vi "Unflatten.vi"(0 "Executioner in":refnum<class "Executioner.lvclass">, 1 "Linked List Ref":refnum<data-value>, 5 "Flattened Test Executive":string, 9 "Linked List ID":string, 11 "error in (no error)":errorcluster, 12 "Persistence in":refnum<class "IPersist.lvclass">, 13 "Compatibility Helper":refnum<class "ICompatibility Helper.lvclass">, 14 "Path Builder":refnum<class "IPath Builder.lvclass">) -> (3 "Linked List Ref out":refnum<data-value>, 6 "Flattened Test Executive out":string, 15 "error out":errorcluster)   [LabVIEW 2020, in "Test Executive.lvlib" / "Executioner.lvclass"]
uses:
  <vilib>/gpm_packages/@cs/test-executive/Source/Test Executive/Executioner/Executioner.lvclass
  <vilib>/gpm_packages/@cs/persistence/source/IPersist/IPersist.lvclass
  <vilib>/gpm_packages/@cs/linked-list/Source/Linked List/ILinkedList/ILinked List.lvclass
  <vilib>/gpm_packages/@cs/test-executive/Source/Path Builder/IPath Builder/IPath Builder.lvclass
  <vilib>/gpm_packages/@cs/test-executive/Source/Compatibility Helper/ICompatibility Helper.lvclass
  7496b3ab-09a6-44dc-ae9e-1065b628b99e.vi
  <vilib>/Utility/error.llb/Error Cluster From Error Code.vi
  <vilib>/ErrorRing/Error Ring.xnode
  <vilib>/gpm_packages/@cs/linked-list/Source/Linked List/Linked List Ref/Linked List Ref.lvclass
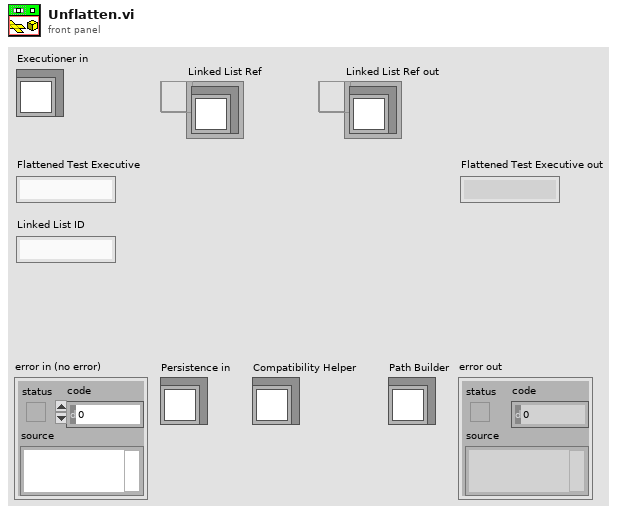
[diagram p1: front panel]
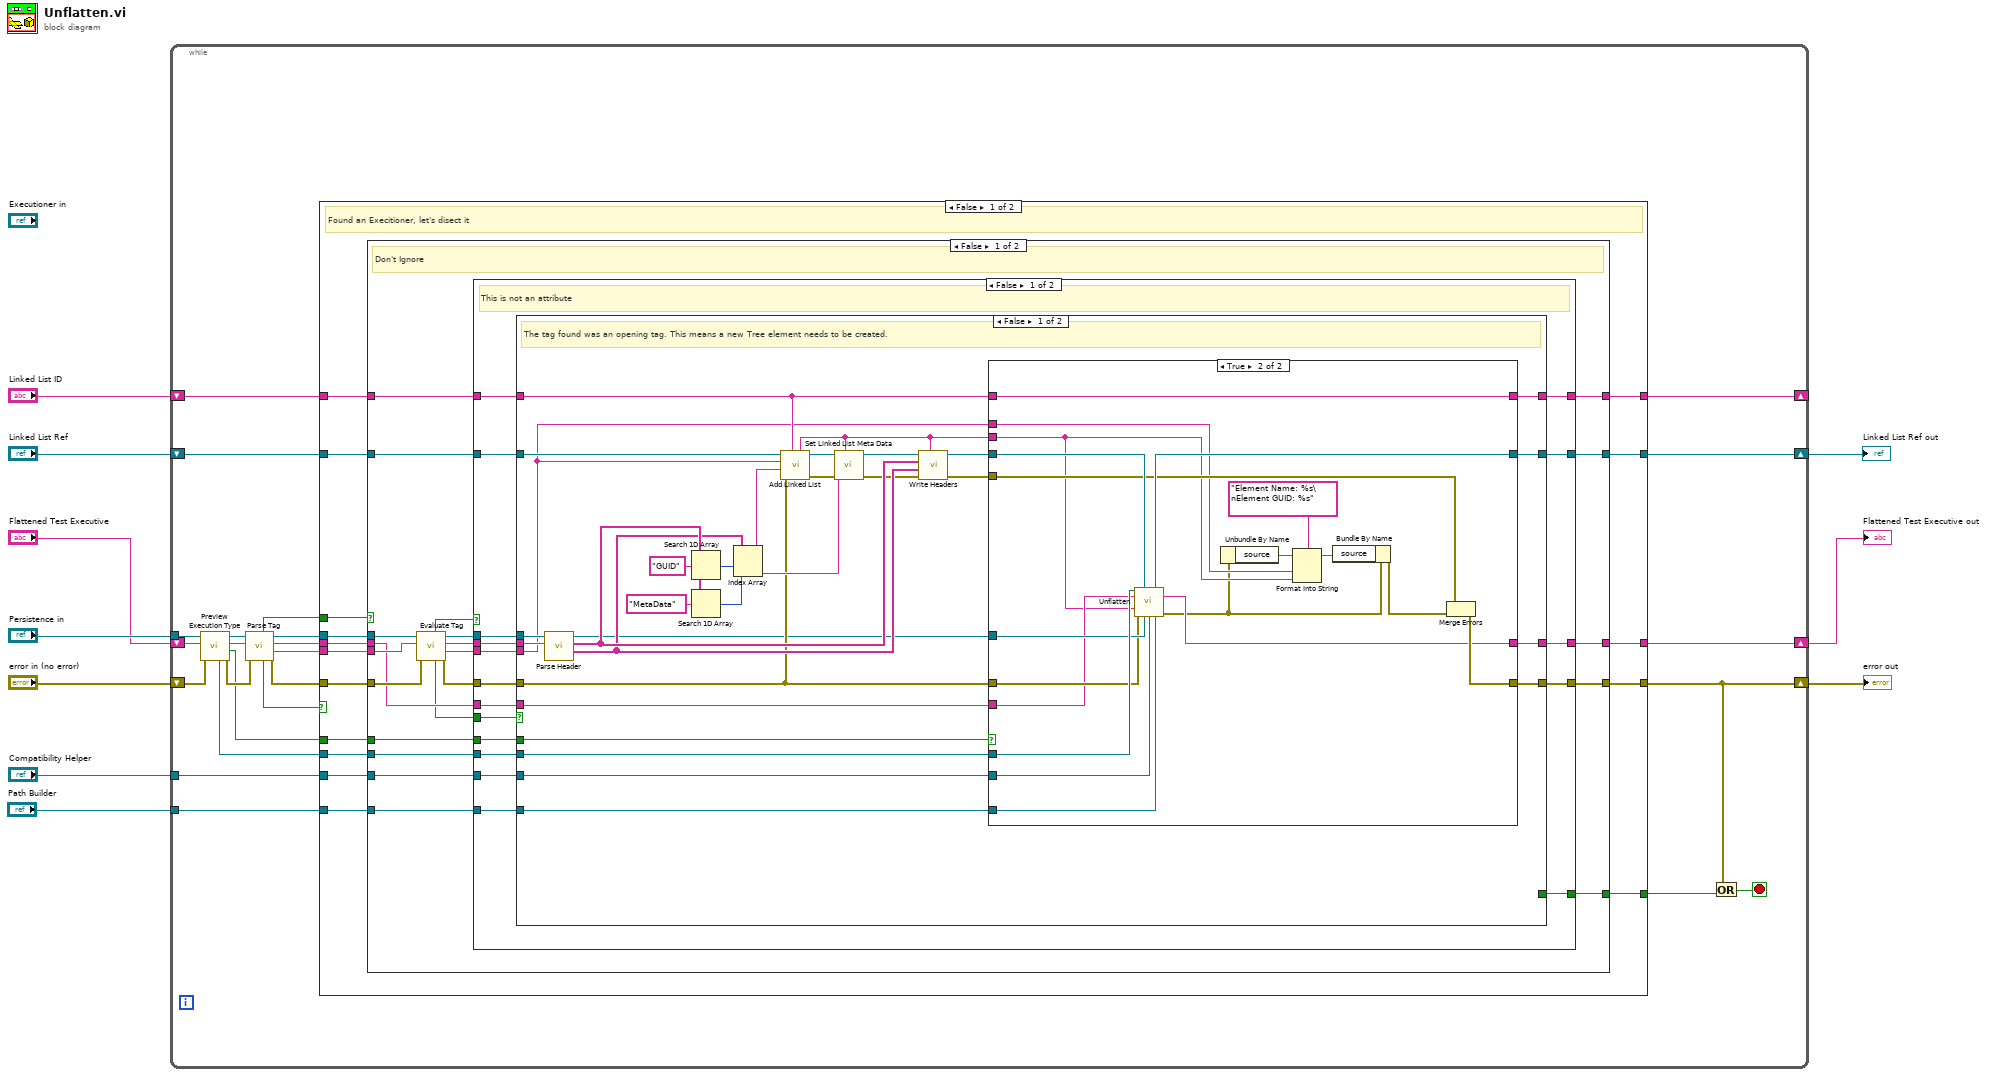
[diagram p0: block diagram]
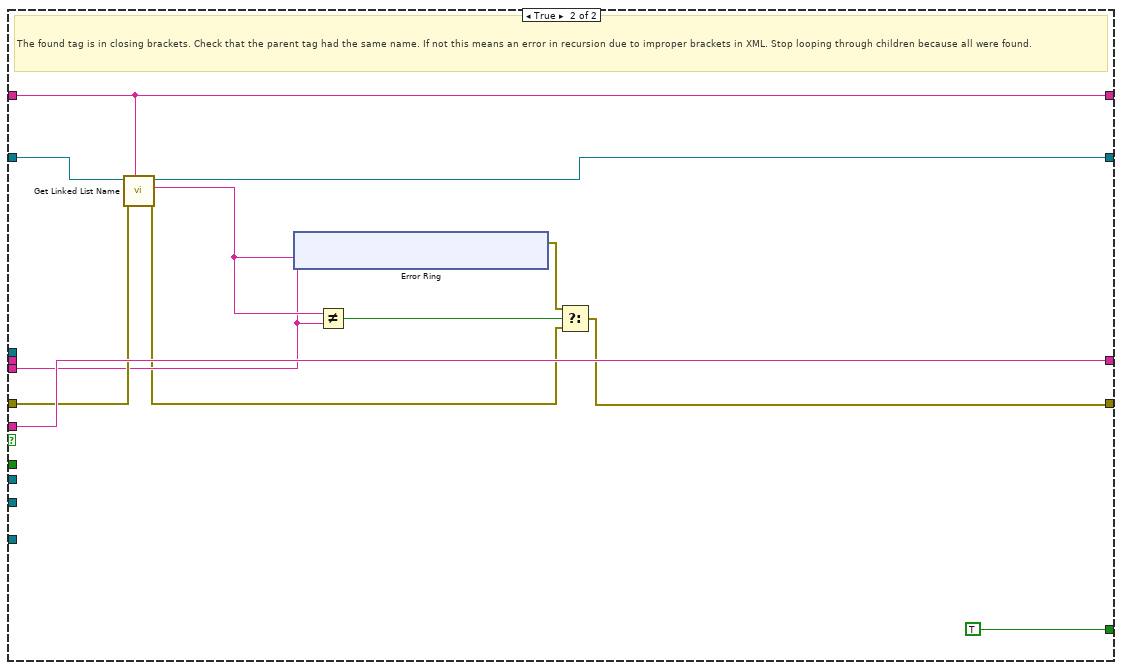
[diagram p3: hidden frame]
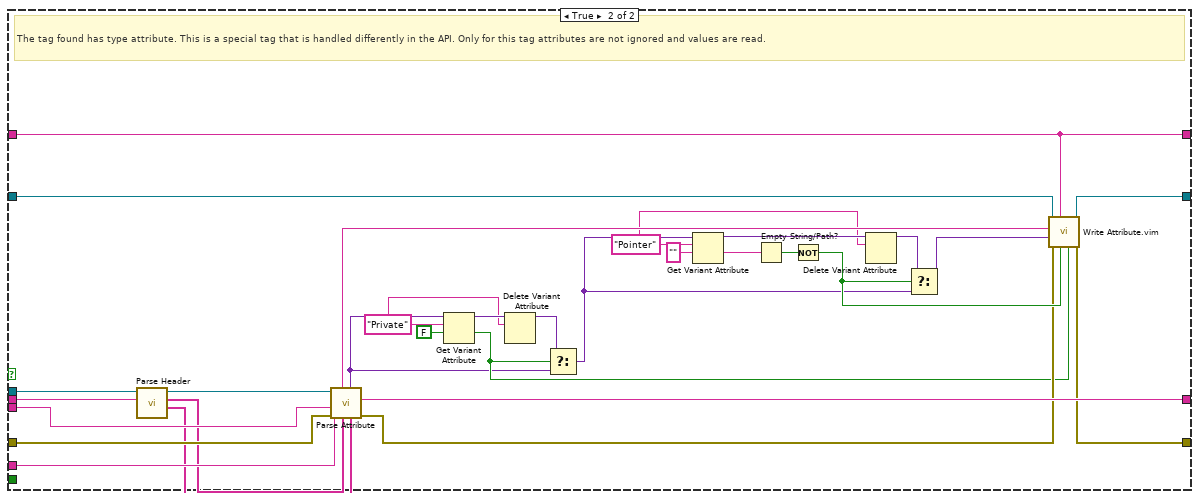
[diagram p4: hidden frame]
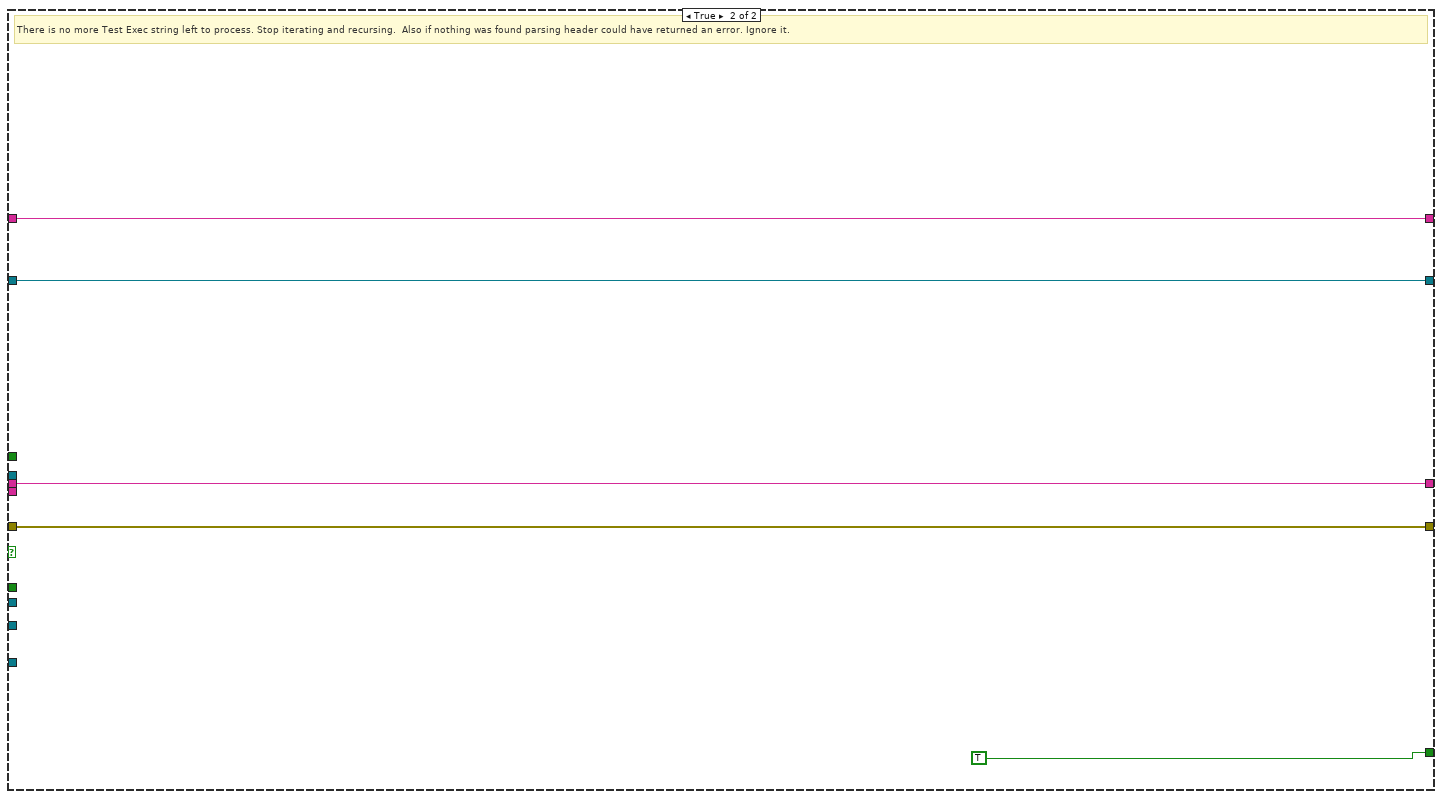
[diagram p6: hidden frame]
diagram:
  n1 = while {
    shift-right: [w32] -> w3
    shift-left: "Flattened Test Executive" -> [w26]
    shift-right: [w11] -> w7
    shift-left: "Linked List Ref" -> [w34]
    shift-right: [w30] -> w4
    shift-left: "error in (no error)" -> [w24]
    shift-right: [w14] -> _
    shift-left: "Linked List ID" -> [w29]
    tunnel: "Persistence in" -> [w28]
    tunnel: "Path Builder" -> [w13]
    tunnel: "Compatibility Helper" -> [w12]
    stop <- w31 stop-if-true
    n2 = call <vilib>:"Preview Execution Type.vi"("error in (no error)"=w24, "Flattened Linked List"=w26, "IPersist in"=w28) -> ("error out"=w23:errorcluster, "Found?"=w16:bool, "Flattened Linked List out"=w25:string, "IPersist out"=w27:refnum<class "IPersist.lvclass">, "Execution Type"=w15:refnum<class "Executioner.lvclass">)  [unwired: 4 in]
    n3 = call-dynamic "Parse Tag.vi"("error in (no error)"=w23, "Flattened Linked List"=w25, "IPersist in"=w27) -> ("error out"=w18:errorcluster, "Tag"=w20:string, "Flattened Linked List After Tag"=w19:string, "IPersist out"=w21:refnum<class "IPersist.lvclass">, "Nothing Found"=w17:bool, "Ignore"=w22:bool)  [unwired: 2 in, 1 out]
    n4 = case shown="False" w17 {
      tunnel: w21 -> [w47 _]
      tunnel: w20 -> [w41 _]
      tunnel: w19 -> [w46 w199]
      tunnel: w18 -> [w43 w198]
      tunnel: w22 -> [w50 _]
      tunnel: w16 -> [w39 _]
      tunnel: w29 -> [w40 w197]
      tunnel: w34 -> [w49 w201]
      tunnel: [w48 w201] -> w11
      tunnel: [w42 TRUE] -> w33
      tunnel: [w45 w199] -> w32
      tunnel: [w44 w198] -> w30
      tunnel: w15 -> [w38 _]
      tunnel: [w37 w197] -> w14
      tunnel: w13 -> [w36 _]
      tunnel: w12 -> [w35 _]
      frame False {
        # "Found an Execitioner, let's disect it"
        n5 = case shown="False" w50 {
          tunnel: w49 -> [w64 w196]
          tunnel: [w56 w196] -> w48
          tunnel: w47 -> [w71 _]
          tunnel: w46 -> [w62 w195]
          tunnel: [w57 w195] -> w45
          tunnel: [w67 w194] -> w44
          tunnel: w43 -> [w69 w194]
          tunnel: [w55 _] -> w42
          tunnel: w41 -> [w70 _]
          tunnel: w40 -> [w63 w193]
          tunnel: w39 -> [w61 _]
          tunnel: w38 -> [w54 _]
          tunnel: [w53 w193] -> w37
          tunnel: w36 -> [w52 _]
          tunnel: w35 -> [w51 _]
          frame False {
            # "Don't Ignore"
            n6 = call-dynamic "Evaluate Tag.vi"("error in (no error)"=w69, "Tag"=w70, "IPersist in"=w71) -> ("error out"=w68:errorcluster, "Tag Name"=w59:string, "Header"=w60:string, "IPersist out"=w65:refnum<class "IPersist.lvclass">, "End of Tag"=w58:bool, "Attribute"=w66:bool)  [unwired: 3 in]
            n7 = case shown="False" w66 {
              tunnel: w68 -> [w83 w187]
              tunnel: [w79 w172] -> w67
              tunnel: w65 -> [w88 w192]
              tunnel: w64 -> [w86 w178]
              tunnel: w63 -> [w74 w171]
              tunnel: w62 -> [w82 w188]
              tunnel: w61 -> [w81 _]
              tunnel: w60 -> [w87 w191]
              tunnel: w59 -> [w84 w189]
              tunnel: w58 -> [w85 _]
              tunnel: [w78 w184] -> w57
              tunnel: [w80 w177] -> w56
              tunnel: [w77 _] -> w55
              tunnel: w54 -> [w76 _]
              tunnel: [w75 w171] -> w53
              tunnel: w52 -> [w73 _]
              tunnel: w51 -> [w72 _]
              frame False {
                # "This is not an attribute"
                n8 = case shown="False" w85 {
                  tunnel: w88 -> [w119 _]
                  tunnel: w87 -> [w118 _]
                  tunnel: w86 -> [w113 w153]
                  tunnel: w84 -> [w89 w146]
                  tunnel: w83 -> [w96 w150]
                  tunnel: w82 -> [w97 w152]
                  tunnel: w81 -> [w98 _]
                  tunnel: w74 -> [w92 w143]
                  tunnel: [w104 w151] -> w80
                  tunnel: [w100 w144] -> w79
                  tunnel: [w99 w152] -> w78
                  tunnel: [_ TRUE] -> w77
                  tunnel: w76 -> [w94 _]
                  tunnel: [w93 w143] -> w75
                  tunnel: w73 -> [w91 _]
                  tunnel: w72 -> [w90 _]
                  frame False {
                    # "The tag found was an opening tag. This means a new Tree element needs to be created."
                    n9 = call-dynamic "Parse Header.vi"("Header"=w118, "IPersist in"=w119) -> ("Value"=w106:string[], "Name"=w107:string[], "IPersist out"=w95:refnum<class "IPersist.lvclass">)  [unwired: 7 in]
                    n10 = Search 1D Array(1D array=w107, element="GUID") -> (index of element=w115:i32)  [unwired: 1 in]
                    n11 = Search 1D Array(1D array=w107, element="MetaData") -> (index of element=w114:i32)  [unwired: 1 in]
                    n12 = Index Array(array=w106, index #1=w115, index #2=w114) -> (element #1=w112:string, element #2=w109:string)
                    n13 = call <vilib>:"Add Linked List.vi"("Parent ID"=w92, "error in (no error)"=w96, "Linked List ID"=w112, "Name"=w89, "Linked List Ref"=w113) -> ("error out"=w110:errorcluster, "Linked List Ref out"=w111:refnum<data-value>, "Linked List ID out"=w102:string)  [unwired: 3 in, 1 out]
                    n14 = call <vilib>:"Set Linked List Meta Data.vi"("Linked List ID"=w102, "error in (no error)"=w110, "Meta Data"=w109, "Linked List Ref"=w111) -> ("error out"=w105:errorcluster, "Linked List Ref out"=w108:refnum<data-value>)  [unwired: 5 in, 1 out]
                    n15 = call <vilib>:"Write Headers.vi"("Linked List ID"=w102, "error in (no error)"=w105, "Header Values"=w106, "Header Names"=w107, "Linked List Ref"=w108) -> ("error out"=w101:errorcluster, "Linked List Ref out"=w103:refnum<data-value>)  [unwired: 5 in]
                    n16 = case shown="True" w98 {
                      tunnel: [w123 w142] -> w104
                      tunnel: w103 -> [w123 w141]
                      tunnel: w102 -> [w120 w128]
                      tunnel: w101 -> [w122 w140]
                      tunnel: [w122 w139] -> w100
                      tunnel: [w121 w138] -> w99
                      tunnel: w95 -> [_ w136]
                      tunnel: w97 -> [w121 w134]
                      tunnel: w96 -> [_ w135]
                      tunnel: w94 -> [_ w137]
                      tunnel: w92 -> [_ w133]
                      tunnel: [w120 w133] -> w93
                      tunnel: w91 -> [_ w132]
                      tunnel: w90 -> [_ w131]
                      tunnel: w89 -> [_ w127]
                      frame False {
                      }
                      frame True {
                        n17 = call-dynamic "Unflatten.vi"("Executioner in"=w137, "Linked List Ref"=w141, "Flattened Test Executive"=w134, "Linked List ID"=w128, "error in (no error)"=w135, "Persistence in"=w136, "Compatibility Helper"=w131, "Path Builder"=w132) -> ("Linked List Ref out"=w142:refnum<data-value>, "Flattened Test Executive out"=w138:string, "error out"=w126:errorcluster)  [unwired: 5 in]
                        n18 = Unbundle By Name(w126) -> ("source"=w130:string)
                        n19 = Format Into String(format string="Element Name: %s\nElement GUID: %s", initial string=w130, w127, w128) -> (resulting string=w124:string)  [unwired: 1 in, 1 out]
                        n20 = Bundle By Name(cluster=w126, "source"=w124) -> (w125:errorcluster)
                        n21 = Merge Errors(w140, w125) -> (w139:errorcluster)
                      }
                    }
                  }
                  frame True {
                    # "The found tag is in closing brackets. Check that the parent tag had the same name. If not this means an error in recursion due to improper brackets in XML. Stop looping through children because all were found."
                    n22 = call <vilib>:"Get Linked List Name.vi"("Linked List ID"=w143, "error in (no error)"=w150, "Linked List Ref"=w153) -> ("error out"=w145:errorcluster, "Linked List Name"=w147:string, "Linked List Ref out"=w151:refnum<data-value>)  [unwired: 5 in, 1 out]
                    n23 = xnode "Error Ring"("parameter 0"=w147, "parameter 1"=w146) -> ("error out"=w148:errorcluster)
                    n24 = Not Equal?(x=w147, y=w146) -> (x != y?=w149:bool)
                    n25 = Select(t=w148, s=w149, f=w145) -> (s? t:f=w144:errorcluster)
                  }
                }
              }
              frame True {
                w164 = "Private" ("name")
                w163 = "Pointer" ("name")
                # "The tag found has type attribute. This is a special tag that is handled differently in the API. Only for this tag attributes are not ignored and values are read."
                n26 = call-dynamic "Parse Header.vi"("Header"=w191, "IPersist in"=w192) -> ("Value"=w185:string[], "Name"=w186:string[], "IPersist out"=w190:refnum<class "IPersist.lvclass">)  [unwired: 7 in]
                n27 = call-dynamic "Parse Attribute.vi"("Header Values"=w185, "Header Names"=w186, "error in (no error)"=w187, "Tag Name"=w189, "Flattened Linked List"=w188, "IPersist in"=w190) -> ("error out"=w173:errorcluster, "Flattened Linked List out"=w184:string, "Attribute Value"=w166:variant, "Attribute Name"=w175:string)  [unwired: 1 in, 1 out]
                n28 = Get Variant Attribute(Variant=w166, name=w164, default value (empty Variant)=FALSE) -> (duplicate Variant=w169:variant, value=w167:bool)  [unwired: 1 in, 2 out]
                n29 = Delete Variant Attribute(6:w164, 7:w169) -> (3:w170:variant)  [unwired: 1 in, 2 out]
                n30 = Select(t=w170, s=w167, f=w166) -> (s? t:f=w165:variant)
                n31 = Get Variant Attribute(Variant=w165, name=w163, default value (empty Variant)="") -> (duplicate Variant=w182:variant, value=w180:string)  [unwired: 1 in, 2 out]
                n32 = Empty String/Path?(string/path=w180) -> (empty?=w179:bool)
                n33 = Not(x=w179) -> (.not. x?=w176:bool)
                n34 = Delete Variant Attribute(6:w163, 7:w182) -> (3:w181:variant)  [unwired: 1 in, 2 out]
                n35 = Select(t=w181, s=w176, f=w165) -> (s? t:f=w174:variant)
                n36 = call "Write Attribute.vim"("Private?"=w167, "Pointer?"=w176, "Linked List ID"=w171, "error in (no error)"=w173, "Attribute"=w174, "Attribute Name"=w175, "Linked List Ref"=w178) -> ("error out"=w172:errorcluster, "Linked List Ref out"=w177:refnum<data-value>)  [unwired: 1 in, 2 out]
              }
            }
          }
          frame True {
            # "Ignore this element due to syntax of header"
          }
        }
      }
      frame True {
        # "There is no more Test Exec string left to process. Stop iterating and recursing.  Also if nothing was found parsing header could have returned an error. Ignore it."
      }
    }
    n37 = Or(x=w30, y=w33) -> (x .or. y?=w31:bool)
  }
  "error out" <- w4
  "Flattened Test Executive out" <- w3
  "Linked List Ref out" <- w7
